vi "Refresh HH Listbox.vi"(5 "AdaptMode":u32, 8 "Command":T1[](array[typedef])=[{"Mode"=enum."Off", "Digital Input"=enum."Unused", "Polarity"=FALSE, "Frequency [Hz]"=0.0, "Duty Cycle [%]"=0.0, "TDC Offset [CAD]"=0.0, "Window Start [DBTDC]"=0.0, "Window End [DBTDC]"=0.0, "Angles"=[{"Enable"=FALSE, "Location [DBTDC]"=0.0, "Duration [s]"=0.0}, {"Enable"=FALSE, "Location [DBTDC]"=0.0, "Duration [s]"=0.0}, {"Enable"=FALSE, "Location [DBTDC]"=0.0, "Duration [s]"=0.0}, {"Enable"=FALSE, "Location [DBTDC]"=0.0, "Duration [s]"=0.0}], "Skip Fire"=FALSE, "Skip Fire Index"=0}, {"Mode"=enum."Off", "Digital Input"=enum."Unused", "Polarity"=FALSE, "Frequency [Hz]"=0.0, "Duty Cycle [%]"=0.0, "TDC Offset [CAD]"=0.0, "Window Start [DBTDC]"=0.0, "Window End [DBTDC]"=0.0, "Angles"=[{"Enable"=FALSE, "Location [DBTDC]"=0.0, "Duration [s]"=0.0}, {"Enable"=FALSE, "Location [DBTDC]"=0.0, "Duration [s]"=0.0}, {"Enable"=FALSE, "Location [DBTDC]"=0.0, "Duration [s]"=0.0}, {"Enable"=FALSE, "Location [DBTDC]"=0.0, "Duration [s]"=0.0}], "Skip Fire"=FALSE, "Skip Fire Index"=0}, {"Mode"=enum."Off", "Digital Input"=enum."Unused", "Polarity"=FALSE, "Frequency [Hz]"=0.0, "Duty Cycle [%]"=0.0, "TDC Offset [CAD]"=0.0, "Window Start [DBTDC]"=0.0, "Window End [DBTDC]"=0.0, "Angles"=[{"Enable"=FALSE, "Location [DBTDC]"=0.0, "Duration [s]"=0.0}, {"Enable"=FALSE, "Location [DBTDC]"=0.0, "Duration [s]"=0.0}, {"Enable"=FALSE, "Location [DBTDC]"=0.0, "Duration [s]"=0.0}, {"Enable"=FALSE, "Location [DBTDC]"=0.0, "Duration [s]"=0.0}], "Skip Fire"=FALSE, "Skip Fire Index"=0}, {"Mode"=enum."Off", "Digital Input"=enum."Unused", "Polarity"=FALSE, "Frequency [Hz]"=0.0, "Duty Cycle [%]"=0.0, "TDC Offset [CAD]"=0.0, "Window Start [DBTDC]"=0.0, "Window End [DBTDC]"=0.0, "Angles"=[{"Enable"=FALSE, "Location [DBTDC]"=0.0, "Duration [s]"=0.0}, {"Enable"=FALSE, "Location [DBTDC]"=0.0, "Duration [s]"=0.0}, {"Enable"=FALSE, "Location [DBTDC]"=0.0, "Duration [s]"=0.0}, {"Enable"=FALSE, "Location [DBTDC]"=0.0, "Duration [s]"=0.0}], "Skip Fire"=FALSE, "Skip Fire Index"=0}, {"Mode"=enum."Off", "Digital Input"=enum."Unused", "Polarity"=FALSE, "Frequency [Hz]"=0.0, "Duty Cycle [%]"=0.0, "TDC Offset [CAD]"=0.0, "Window Start [DBTDC]"=0.0, "Window End [DBTDC]"=0.0, "Angles"=[{"Enable"=FALSE, "Location [DBTDC]"=0.0, "Duration [s]"=0.0}, {"Enable"=FALSE, "Location [DBTDC]"=0.0, "Duration [s]"=0.0}, {"Enable"=FALSE, "Location [DBTDC]"=0.0, "Duration [s]"=0.0}, {"Enable"=FALSE, "Location [DBTDC]"=0.0, "Duration [s]"=0.0}], "Skip Fire"=FALSE, "Skip Fire Index"=0}, {"Mode"=enum."Off", "Digital Input"=enum."Unused", "Polarity"=FALSE, "Frequency [Hz]"=0.0, "Duty Cycle [%]"=0.0, "TDC Offset [CAD]"=0.0, "Window Start [DBTDC]"=0.0, "Window End [DBTDC]"=0.0, "Angles"=[{"Enable"=FALSE, "Location [DBTDC]"=0.0, "Duration [s]"=0.0}, {"Enable"=FALSE, "Location [DBTDC]"=0.0, "Duration [s]"=0.0}, {"Enable"=FALSE, "Location [DBTDC]"=0.0, "Duration [s]"=0.0}, {"Enable"=FALSE, "Location [DBTDC]"=0.0, "Duration [s]"=0.0}], "Skip Fire"=FALSE, "Skip Fire Index"=0}, {"Mode"=enum."Off", "Digital Input"=enum."Unused", "Polarity"=FALSE, "Frequency [Hz]"=0.0, "Duty Cycle [%]"=0.0, "TDC Offset [CAD]"=0.0, "Window Start [DBTDC]"=0.0, "Window End [DBTDC]"=0.0, "Angles"=[{"Enable"=FALSE, "Location [DBTDC]"=0.0, "Duration [s]"=0.0}, {"Enable"=FALSE, "Location [DBTDC]"=0.0, "Duration [s]"=0.0}, {"Enable"=FALSE, "Location [DBTDC]"=0.0, "Duration [s]"=0.0}, {"Enable"=FALSE, "Location [DBTDC]"=0.0, "Duration [s]"=0.0}], "Skip Fire"=FALSE, "Skip Fire Index"=0}, {"Mode"=enum."Off", "Digital Input"=enum."Unused", "Polarity"=FALSE, "Frequency [Hz]"=0.0, "Duty Cycle [%]"=0.0, "TDC Offset [CAD]"=0.0, "Window Start [DBTDC]"=0.0, "Window End [DBTDC]"=0.0, "Angles"=[{"Enable"=FALSE, "Location [DBTDC]"=0.0, "Duration [s]"=0.0}, {"Enable"=FALSE, "Location [DBTDC]"=0.0, "Duration [s]"=0.0}, {"Enable"=FALSE, "Location [DBTDC]"=0.0, "Duration [s]"=0.0}, {"Enable"=FALSE, "Location [DBTDC]"=0.0, "Duration [s]"=0.0}], "Skip Fire"=FALSE, "Skip Fire Index"=0}] {"Skip Fire Index" max=7; "Angles"."Duration [s]" format="%#_3p"; "Frequency [Hz]" format="%#_3p"}, 9 "Names":string[](array[string]), 10 "Config":T5[](array[typedef]) {"ISeq"."Duration [s]" min=0 max=26 format="%#_3p"; "ISeq"."Lower [A]" min=0 max=8 format="%#_3p"; "ISeq"."Upper [A]" min=0 max=8 format="%#_3p"}, 11 "_Listbox":refnum<vi>) -> (0 "Command out":T1[](array[typedef])=[{"Mode"=enum."Off", "Digital Input"=enum."Unused", "Polarity"=FALSE, "Frequency [Hz]"=0.0, "Duty Cycle [%]"=0.0, "TDC Offset [CAD]"=0.0, "Window Start [DBTDC]"=0.0, "Window End [DBTDC]"=0.0, "Angles"=[{"Enable"=FALSE, "Location [DBTDC]"=0.0, "Duration [s]"=0.0}, {"Enable"=FALSE, "Location [DBTDC]"=0.0, "Duration [s]"=0.0}, {"Enable"=FALSE, "Location [DBTDC]"=0.0, "Duration [s]"=0.0}, {"Enable"=FALSE, "Location [DBTDC]"=0.0, "Duration [s]"=0.0}], "Skip Fire"=FALSE, "Skip Fire Index"=0}, {"Mode"=enum."Off", "Digital Input"=enum."Unused", "Polarity"=FALSE, "Frequency [Hz]"=0.0, "Duty Cycle [%]"=0.0, "TDC Offset [CAD]"=0.0, "Window Start [DBTDC]"=0.0, "Window End [DBTDC]"=0.0, "Angles"=[{"Enable"=FALSE, "Location [DBTDC]"=0.0, "Duration [s]"=0.0}, {"Enable"=FALSE, "Location [DBTDC]"=0.0, "Duration [s]"=0.0}, {"Enable"=FALSE, "Location [DBTDC]"=0.0, "Duration [s]"=0.0}, {"Enable"=FALSE, "Location [DBTDC]"=0.0, "Duration [s]"=0.0}], "Skip Fire"=FALSE, "Skip Fire Index"=0}, {"Mode"=enum."Off", "Digital Input"=enum."Unused", "Polarity"=FALSE, "Frequency [Hz]"=0.0, "Duty Cycle [%]"=0.0, "TDC Offset [CAD]"=0.0, "Window Start [DBTDC]"=0.0, "Window End [DBTDC]"=0.0, "Angles"=[{"Enable"=FALSE, "Location [DBTDC]"=0.0, "Duration [s]"=0.0}, {"Enable"=FALSE, "Location [DBTDC]"=0.0, "Duration [s]"=0.0}, {"Enable"=FALSE, "Location [DBTDC]"=0.0, "Duration [s]"=0.0}, {"Enable"=FALSE, "Location [DBTDC]"=0.0, "Duration [s]"=0.0}], "Skip Fire"=FALSE, "Skip Fire Index"=0}, {"Mode"=enum."Off", "Digital Input"=enum."Unused", "Polarity"=FALSE, "Frequency [Hz]"=0.0, "Duty Cycle [%]"=0.0, "TDC Offset [CAD]"=0.0, "Window Start [DBTDC]"=0.0, "Window End [DBTDC]"=0.0, "Angles"=[{"Enable"=FALSE, "Location [DBTDC]"=0.0, "Duration [s]"=0.0}, {"Enable"=FALSE, "Location [DBTDC]"=0.0, "Duration [s]"=0.0}, {"Enable"=FALSE, "Location [DBTDC]"=0.0, "Duration [s]"=0.0}, {"Enable"=FALSE, "Location [DBTDC]"=0.0, "Duration [s]"=0.0}], "Skip Fire"=FALSE, "Skip Fire Index"=0}, {"Mode"=enum."Off", "Digital Input"=enum."Unused", "Polarity"=FALSE, "Frequency [Hz]"=0.0, "Duty Cycle [%]"=0.0, "TDC Offset [CAD]"=0.0, "Window Start [DBTDC]"=0.0, "Window End [DBTDC]"=0.0, "Angles"=[{"Enable"=FALSE, "Location [DBTDC]"=0.0, "Duration [s]"=0.0}, {"Enable"=FALSE, "Location [DBTDC]"=0.0, "Duration [s]"=0.0}, {"Enable"=FALSE, "Location [DBTDC]"=0.0, "Duration [s]"=0.0}, {"Enable"=FALSE, "Location [DBTDC]"=0.0, "Duration [s]"=0.0}], "Skip Fire"=FALSE, "Skip Fire Index"=0}, {"Mode"=enum."Off", "Digital Input"=enum."Unused", "Polarity"=FALSE, "Frequency [Hz]"=0.0, "Duty Cycle [%]"=0.0, "TDC Offset [CAD]"=0.0, "Window Start [DBTDC]"=0.0, "Window End [DBTDC]"=0.0, "Angles"=[{"Enable"=FALSE, "Location [DBTDC]"=0.0, "Duration [s]"=0.0}, {"Enable"=FALSE, "Location [DBTDC]"=0.0, "Duration [s]"=0.0}, {"Enable"=FALSE, "Location [DBTDC]"=0.0, "Duration [s]"=0.0}, {"Enable"=FALSE, "Location [DBTDC]"=0.0, "Duration [s]"=0.0}], "Skip Fire"=FALSE, "Skip Fire Index"=0}, {"Mode"=enum."Off", "Digital Input"=enum."Unused", "Polarity"=FALSE, "Frequency [Hz]"=0.0, "Duty Cycle [%]"=0.0, "TDC Offset [CAD]"=0.0, "Window Start [DBTDC]"=0.0, "Window End [DBTDC]"=0.0, "Angles"=[{"Enable"=FALSE, "Location [DBTDC]"=0.0, "Duration [s]"=0.0}, {"Enable"=FALSE, "Location [DBTDC]"=0.0, "Duration [s]"=0.0}, {"Enable"=FALSE, "Location [DBTDC]"=0.0, "Duration [s]"=0.0}, {"Enable"=FALSE, "Location [DBTDC]"=0.0, "Duration [s]"=0.0}], "Skip Fire"=FALSE, "Skip Fire Index"=0}, {"Mode"=enum."Off", "Digital Input"=enum."Unused", "Polarity"=FALSE, "Frequency [Hz]"=0.0, "Duty Cycle [%]"=0.0, "TDC Offset [CAD]"=0.0, "Window Start [DBTDC]"=0.0, "Window End [DBTDC]"=0.0, "Angles"=[{"Enable"=FALSE, "Location [DBTDC]"=0.0, "Duration [s]"=0.0}, {"Enable"=FALSE, "Location [DBTDC]"=0.0, "Duration [s]"=0.0}, {"Enable"=FALSE, "Location [DBTDC]"=0.0, "Duration [s]"=0.0}, {"Enable"=FALSE, "Location [DBTDC]"=0.0, "Duration [s]"=0.0}], "Skip Fire"=FALSE, "Skip Fire Index"=0}] {"Skip Fire Index" max=7; "Angles"."Duration [s]" format="%#_3p"; "Frequency [Hz]" format="%#_3p"}, 2 "Config out":T5[](array[typedef]) {"ISeq"."Duration [s]" min=0 max=26 format="%#_3p"; "ISeq"."Lower [A]" min=0 max=8 format="%#_3p"; "ISeq"."Upper [A]" min=0 max=8 format="%#_3p"}, 4 "AdaptMode":u32, 6 "Disabled Configs":i32[](array[numeric]))   [LabVIEW 2016]
uses:
  <vilib>/Powertrain Controls/Device Drivers/DCM/HH/RT/Config.ctl
  <vilib>/Powertrain Controls/Device Drivers/DCM/HH/RT/Mode.ctl
  <vilib>/Powertrain Controls/Device Drivers/DCM/HH/RT/ISeq.ctl
  <vilib>/Powertrain Controls/Device Drivers/DCM/HH/RT/Setup.ctl
  <vilib>/Powertrain Controls/Device Drivers/DCM/HH/FPGA/Mode.ctl
  <vilib>/Powertrain Controls/Device Drivers/DCM/Rev0/FPGA/Digital Channel.ctl
  <vilib>/Powertrain Controls/Device Drivers/DCM/HH/RT/Angle Control.ctl
  <vilib>/Powertrain Controls/Device Drivers/DCM/HH/RT/DCM - RT - HH.lvlib
  <vilib>/Powertrain Controls/Device Drivers/DCM/HH/FPGA/DCM - FPGA - HH.lvlib
  <vilib>/Powertrain Controls/Device Drivers/DCM/Rev0/FPGA/DCM - FPGA.lvlib
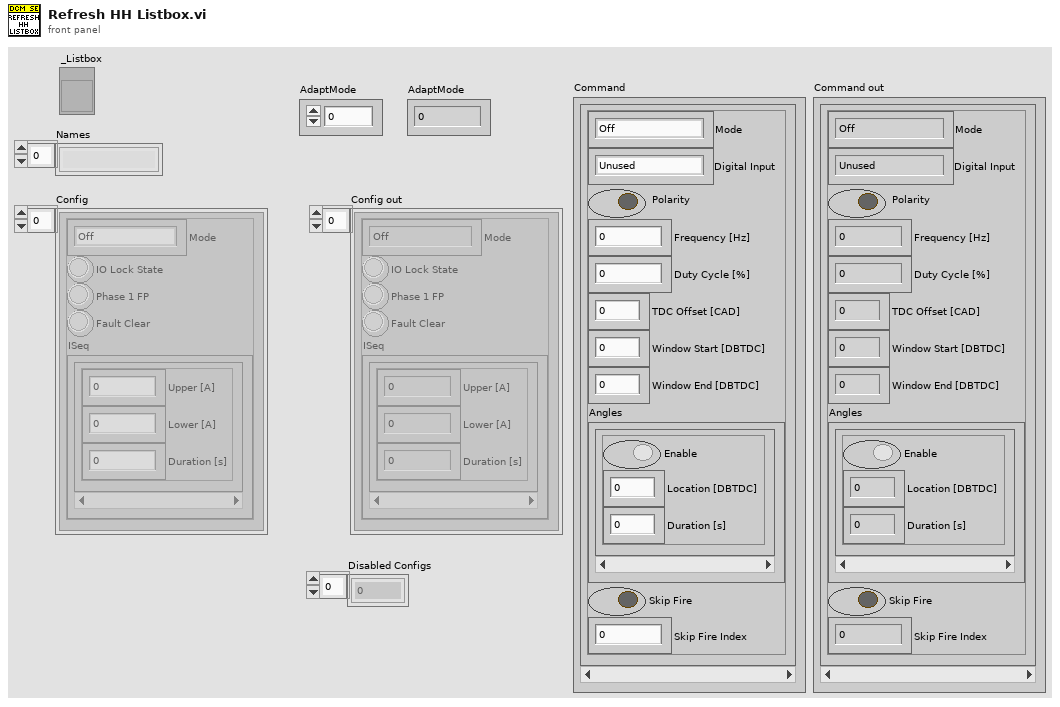
[diagram p1: front panel]
types:
  T1 = typedef "DCM - RT - HH.lvlib/Setup.ctl" = cluster{"Mode":T2, "Digital Input":T3, "Polarity":bool, "Frequency [Hz]":sgl, "Duty Cycle [%]":sgl, "TDC Offset [CAD]":sgl, "Window Start [DBTDC]":sgl, "Window End [DBTDC]":sgl, "Angles":T4[], "Skip Fire":bool, "Skip Fire Index":u8}
  T2 = typedef "DCM - FPGA - HH.lvlib/Mode.ctl" = enum8{"Off", "Direct", "Pulse Width Modulation", "Engine Position Tracking"}
  T3 = typedef "DCM - FPGA.lvlib/Digital Channel.ctl" = enum8{"Unused", "User OS", "Diff IO 1", "Diff IO 2", "Diff IO 3", "Diff IO 4", "Diff IO 5", "Diff IO 6", "Diff IO 7", "Diff IO 8", "Aux 1", "Aux 2", "Aux 3", "Aux 4", "Aux 5", "Aux 6", "Aux 7", "Aux 8", "Aux 9", "Aux 10", "Aux 11", "Aux 12", "Aux 13", "Aux 14", "Aux 15", "Aux 16"}
  T4 = typedef "DCM - RT - HH.lvlib/Angle Control.ctl" = cluster{"Enable":bool, "Location [DBTDC]":sgl, "Duration [s]":sgl}
  T5 = typedef "DCM - RT - HH.lvlib/Config.ctl" = cluster{"Mode":T6, "IO Lock State":bool, "Phase 1 FP":bool, "Fault Clear":bool, "ISeq":T7[]}
  T6 = typedef "DCM - RT - HH.lvlib/Mode.ctl" = enum16{"Off", "Lowside", "Highside", "PFI", "Full H", "3-Phase"}
  T7 = typedef "DCM - RT - HH.lvlib/ISeq.ctl" = cluster{"Upper [A]":sgl, "Lower [A]":sgl, "Duration [s]":sgl}
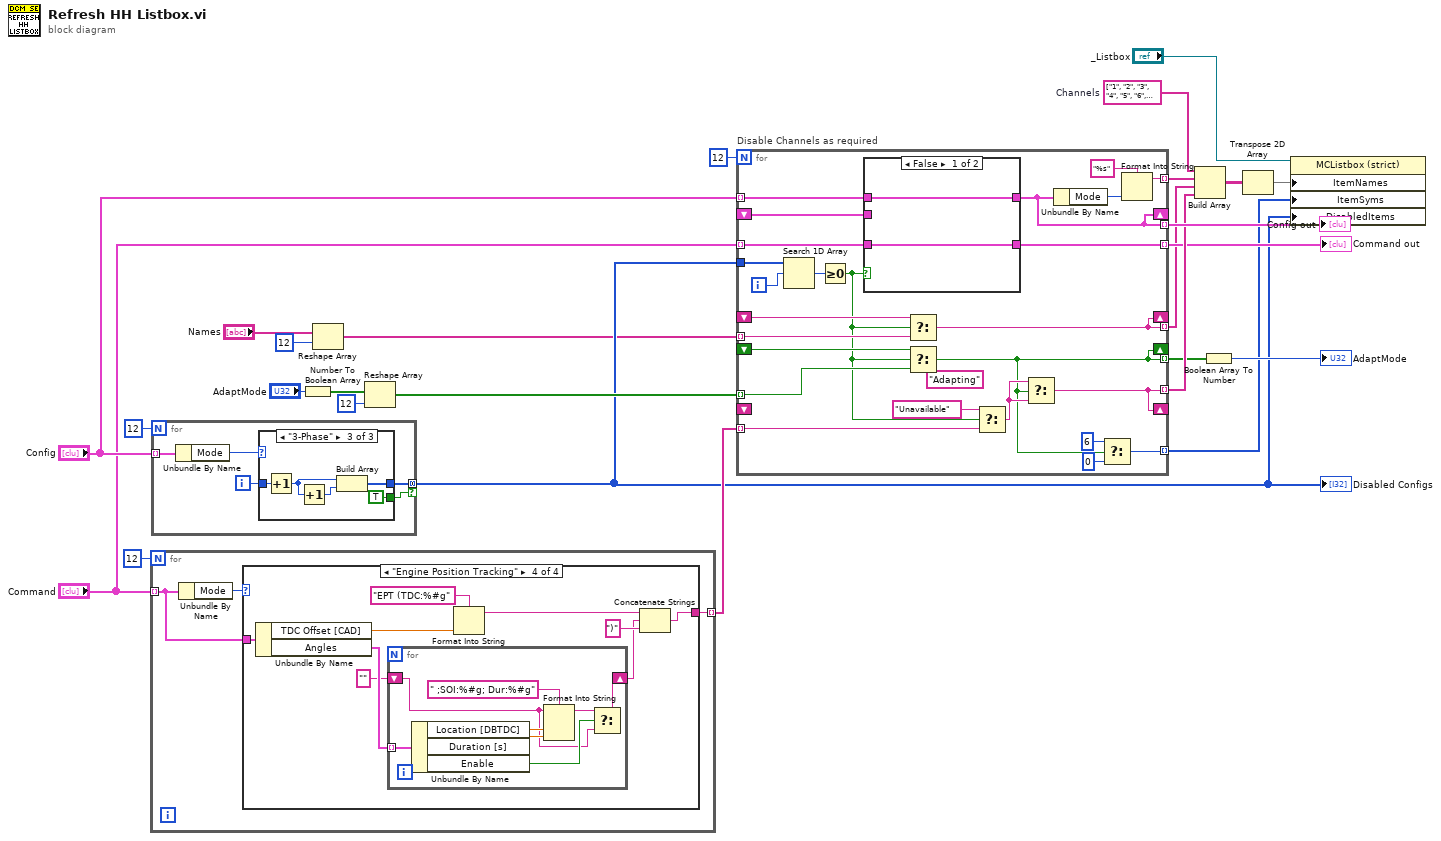
[diagram p0: block diagram]
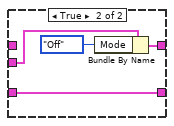
[diagram p2: hidden frame]
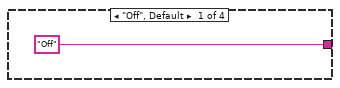
[diagram p3: hidden frame]
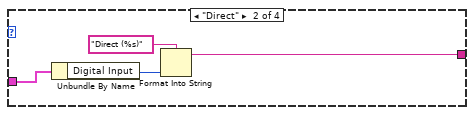
[diagram p4: hidden frame]
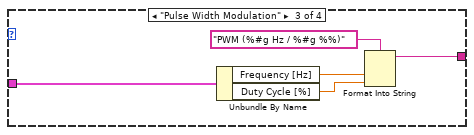
[diagram p5: hidden frame]
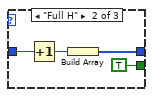
[diagram p7: hidden frame]
diagram:
  w24 = string[] ["1", "2", "3", "4", "5", "6", "7", "8", "9", "10", "11", "12"]  # Channels
  n1 = for {
    N: 12 -> [_]
    tunnel: "Command" -> [w28] mode=indexing
    tunnel: [w27] -> w19 mode=indexing
    n2 = Unbundle By Name(w28) -> ("Mode"=w29:T2)
    n3 = case shown="\"Engine Position Tracking\"" w29 {
      tunnel: w28 -> [_ w34 w39 w47]
      tunnel: ["Off" w31 w35 w43] -> w27
      frame "Off", Default {
      }
      frame "Direct" {
        n4 = Unbundle By Name(w34) -> ("Digital Input"=w32:T3)
        n5 = Format Into String(format string="Direct (%s)", w32) -> (resulting string=w31:string)  [unwired: 2 in, 1 out]
      }
      frame "Pulse Width Modulation" {
        n6 = Unbundle By Name(w39) -> ("Frequency [Hz]"=w37:sgl, "Duty Cycle [%]"=w36:sgl)
        n7 = Format Into String(format string="PWM (%#g Hz / %#g %%)", w37, w36) -> (resulting string=w35:string)  [unwired: 2 in, 1 out]
      }
      frame "Engine Position Tracking" {
        n8 = Unbundle By Name(w47) -> ("TDC Offset [CAD]"=w46:sgl, "Angles"=w45:T4[])
        n9 = for {
          tunnel: w45 -> [w54] mode=indexing
          shift-right: [w50] -> w41
          shift-left: "" -> [w49]
          n10 = Unbundle By Name(w54) -> ("Location [DBTDC]"=w55:sgl, "Duration [s]"=w53:sgl, "Enable"=w52:bool)
          n11 = Format Into String(format string=" ;SOI:%#g; Dur:%#g", initial string=w49, w55, w53) -> (resulting string=w51:string)  [unwired: 1 in, 1 out]
          n12 = Select(t=w51, s=w52, f=w49) -> (s? t:f=w50:string)
        }
        n13 = Format Into String(format string="EPT (TDC:%#g", w46) -> (resulting string=w44:string)  [unwired: 2 in, 1 out]
        n14 = Concatenate Strings(w44, w41, ")" ("string")) -> (w43:string)
      }
    }
  }
  n15 = for {
    N: 12 -> [_]
    tunnel: "Config" -> [w61] mode=indexing
    tunnel: [w58] -> w5 mode=concatenating if=w57
    i -> [w59]
    n16 = Unbundle By Name(w61) -> ("Mode"=w60:T6)
    n17 = case shown="\"3-Phase\"" w60 {
      tunnel: w59 -> [_ w65 w70]
      tunnel: [_ w64 w67] -> w58
      tunnel: [_ TRUE TRUE] -> w57
      frame "Off", Default {
      }
      frame "Full H" {
        n18 = Increment(x=w65) -> (x+1=w63:i32)
        n19 = Build Array(w63) -> (w64:i32[])
      }
      frame "3-Phase" {
        n20 = Increment(x=w70) -> (x+1=w69:i32)
        n21 = Increment(x=w69) -> (x+1=w68:i32)
        n22 = Build Array(w69, w68) -> (w67:i32[])
      }
    }
  }
  "Disabled Configs" <- w5
  n23 = Number To Boolean Array(number="AdaptMode") -> (Boolean array=w10:bool[])
  n24 = Reshape Array("Names", 12 ("dimension size")) -> (w4:string[])
  n25 = Reshape Array(w10, 12 ("dimension size")) -> (w8:bool[])
  n26 = for "Disable Channels as required" {
    N: 12 -> [_]
    tunnel: "Config" -> [w89] mode=indexing
    tunnel: w5 -> [w95]
    tunnel: [w72] -> w20 mode=indexing
    tunnel: [w90] -> w21 mode=indexing
    tunnel: w19 -> [w85] mode=indexing
    tunnel: [w80] -> w18 mode=indexing
    tunnel: [w87] -> w17 mode=indexing
    tunnel: "Command" -> [w88] mode=indexing
    tunnel: w8 -> [w84] mode=indexing
    tunnel: [w74] -> w7 mode=indexing
    tunnel: w4 -> [w86] mode=indexing
    tunnel: [w83] -> w3 mode=indexing
    shift-right: [w83] -> _
    shift-left: _ -> [w82]
    shift-right: [w74] -> _
    shift-left: _ -> [w81]
    shift-right: [w80] -> _
    shift-left: _ -> [_]
    tunnel: [w79] -> w2 mode=indexing
    shift-right: [w72] -> _
    shift-left: _ -> [w71]
    i -> [w94]
    (unwired) "Adapting" ("format string")
    n27 = Search 1D Array(1D array=w95, element=w94) -> (index of element=w93:i32)  [unwired: 1 in]
    n28 = Greater Or Equal To 0?(x=w93) -> (x >= 0?=w77:bool)
    n29 = case shown="False" w77 {
      tunnel: w89 -> [w97 _]
      tunnel: [w97 w100] -> w72
      tunnel: w88 -> [w96 w101]
      tunnel: [w96 w101] -> w87
      tunnel: w71 -> [_ w98]
      frame False {
      }
      frame True {
        n30 = Bundle By Name(cluster=w98, "Mode"=Mode."Off") -> (w100:T5)
      }
    }
    n31 = Select(t=w82, s=w77, f=w86) -> (s? t:f=w83:string)
    n32 = Select(t=w81, s=w77, f=w84) -> (s? t:f=w74:bool)
    n33 = Select(t="Unavailable", s=w77, f=w85) -> (s? t:f=w76:string)
    n34 = Select(t=w76, s=w74, f=w76) -> (s? t:f=w80:string)
    n35 = Unbundle By Name(w72) -> ("Mode"=w91:T6)
    n36 = Select(t=6, s=w74, f=0) -> (s? t:f=w79:i32)
    n37 = Format Into String(format string="%s", w91) -> (resulting string=w90:string)  [unwired: 2 in, 1 out]
  }
  "Config out" <- w20
  "Command out" <- w17
  n38 = Build Array(w24, w21, w3, w18) -> (w26:string[][])
  n39 = Boolean Array To Number(Boolean array=w7) -> (number=→"AdaptMode":u32)
  n40 = Transpose 2D Array(2D array=w26) -> (transposed array=w23:string[][])
  n41 = property on="Property Node" class="MCListbox (strict)"(reference="_Listbox", "ItemNames"=w23, "ItemSyms"=w2, "DisabledItems"=w5) -> ()  [unwired: 1 in, 2 out]
